vi "SpectrumCursor_readGroups.vi"(1 "first 4 letters from\ncursors group name":string="poly", 2 "graph ref":refnum<vi>) -> (0 "cursors\npositions":cluster{"X":dbl, "Y":dbl}[](array[cluster]))   [LabVIEW 2010]
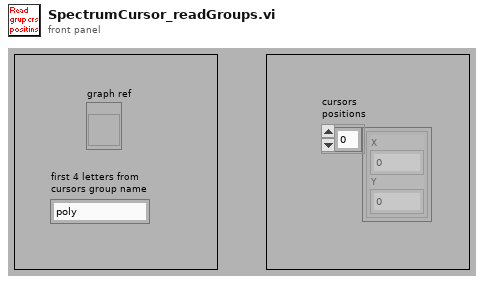
[diagram p1: front panel]
types:
  T1 = typedef "LVCursorListTypeDef.ctl" = cluster{"Name":string, "Color":u32, "Style":u8, "Point Style":u8, "Name Visible":bool, "Allow Drag":bool, "Cursor Mode":u32, "Plot":i32, "Index":i32, "Position":cluster{"X":dbl, "Y":dbl}, "X Scale":u32, "Y Scale":u32, "Watch Plots":i32[], "Watch All Plots":bool, "Plot Area":i32, "Label Offset":cluster{"X":dbl, "Y":dbl}}[]
  T2 = cluster{"Name":string, "Color":u32, "Style":u8, "Point Style":u8, "Name Visible":bool, "Allow Drag":bool, "Cursor Mode":u32, "Plot":i32, "Index":i32, "Position":cluster{"X":dbl, "Y":dbl}, "X Scale":u32, "Y Scale":u32, "Watch Plots":i32[], "Watch All Plots":bool, "Plot Area":i32, "Label Offset":cluster{"X":dbl, "Y":dbl}}
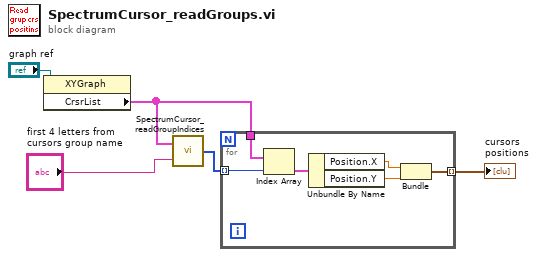
[diagram p0: block diagram]
diagram:
  n1 = property class="XYGraph"(reference="graph ref") -> ("CrsrList"=w2:T1)  [unwired: 1 in, 2 out]
  n2 = call "SpectrumCursor_readGroupIndices.vi"("first 4 letters\nfrom cursor\nname"="first 4 letters from\ncursors group name", "Cursor List"=w2) -> ("cursors\nindeces"=w4:i32[])
  n3 = for {
    tunnel: w2 -> [w10]
    tunnel: w4 -> [w9] mode=indexing
    tunnel: [w6] -> w1 mode=indexing
    n4 = Index Array(array=w10, index=w9) -> (element=w11:T2)
    n5 = Unbundle By Name(w11) -> ("Position.X"=w7:dbl, "Position.Y"=w8:dbl)
    n6 = Bundle("X"=w7, "Y"=w8) -> (w6:cluster{"X":dbl, "Y":dbl})  [unwired: 1 in]
  }
  "cursors\npositions" <- w1
